vi "State Config.vi"(10 "stations count":i32=1, 11 "configuration file path":path) -> (0 "error out":errorcluster, 3 "all state configs":T4[](array[typedef]))   [LabVIEW 2018]
uses:
  Crl defs/DataStream.ctl
  Crl defs/one state paths config.ctl
  Crl defs/one state prints config.ctl
  Communication connection/Crl defs/print config.ctl
  Crl defs/one state scans config.ctl
  Communication connection/Crl defs/scanner config.ctl
  Crl defs/one state tags config.ctl
  Crl defs/PLC_bool tags.ctl
  DataSocket/Crl defs/DataSocket_Tags.ctl
  Crl defs/PLC_real tags.ctl
  Crl defs/PLC_string tags.ctl
  Crl defs/one state msic config.ctl
  Sequence/type defs/Sequence Info.ctl
  Crl defs/one state power supply config.ctl
  Crl defs/motor operating data.ctl
  Crl defs/one state screw config.ctl
  Crl defs/xls.data'S buffer.ctl
  Crl defs/XLS.header configs.ctl
  Interface/Crl defs/HomeScreens.ctl
  Interface/Crl defs/HomeScreen.ctl
  Interface/Crl defs/StatusBars.ctl
panel:
  out "HomeScreens":T1 {"Database LVDT's Data Out"."value" format="%.2f"; "StatusBar"."Cycle Time Br" format="%#_5g"}
  # "Pass / Fail"
  # "Station"
  # "Barcode"
  # "Barcode OK?"
  # "Ser Number"
  # "Part Type"
  # "Application Status"
  # "Cycle Time"
  # "Time"
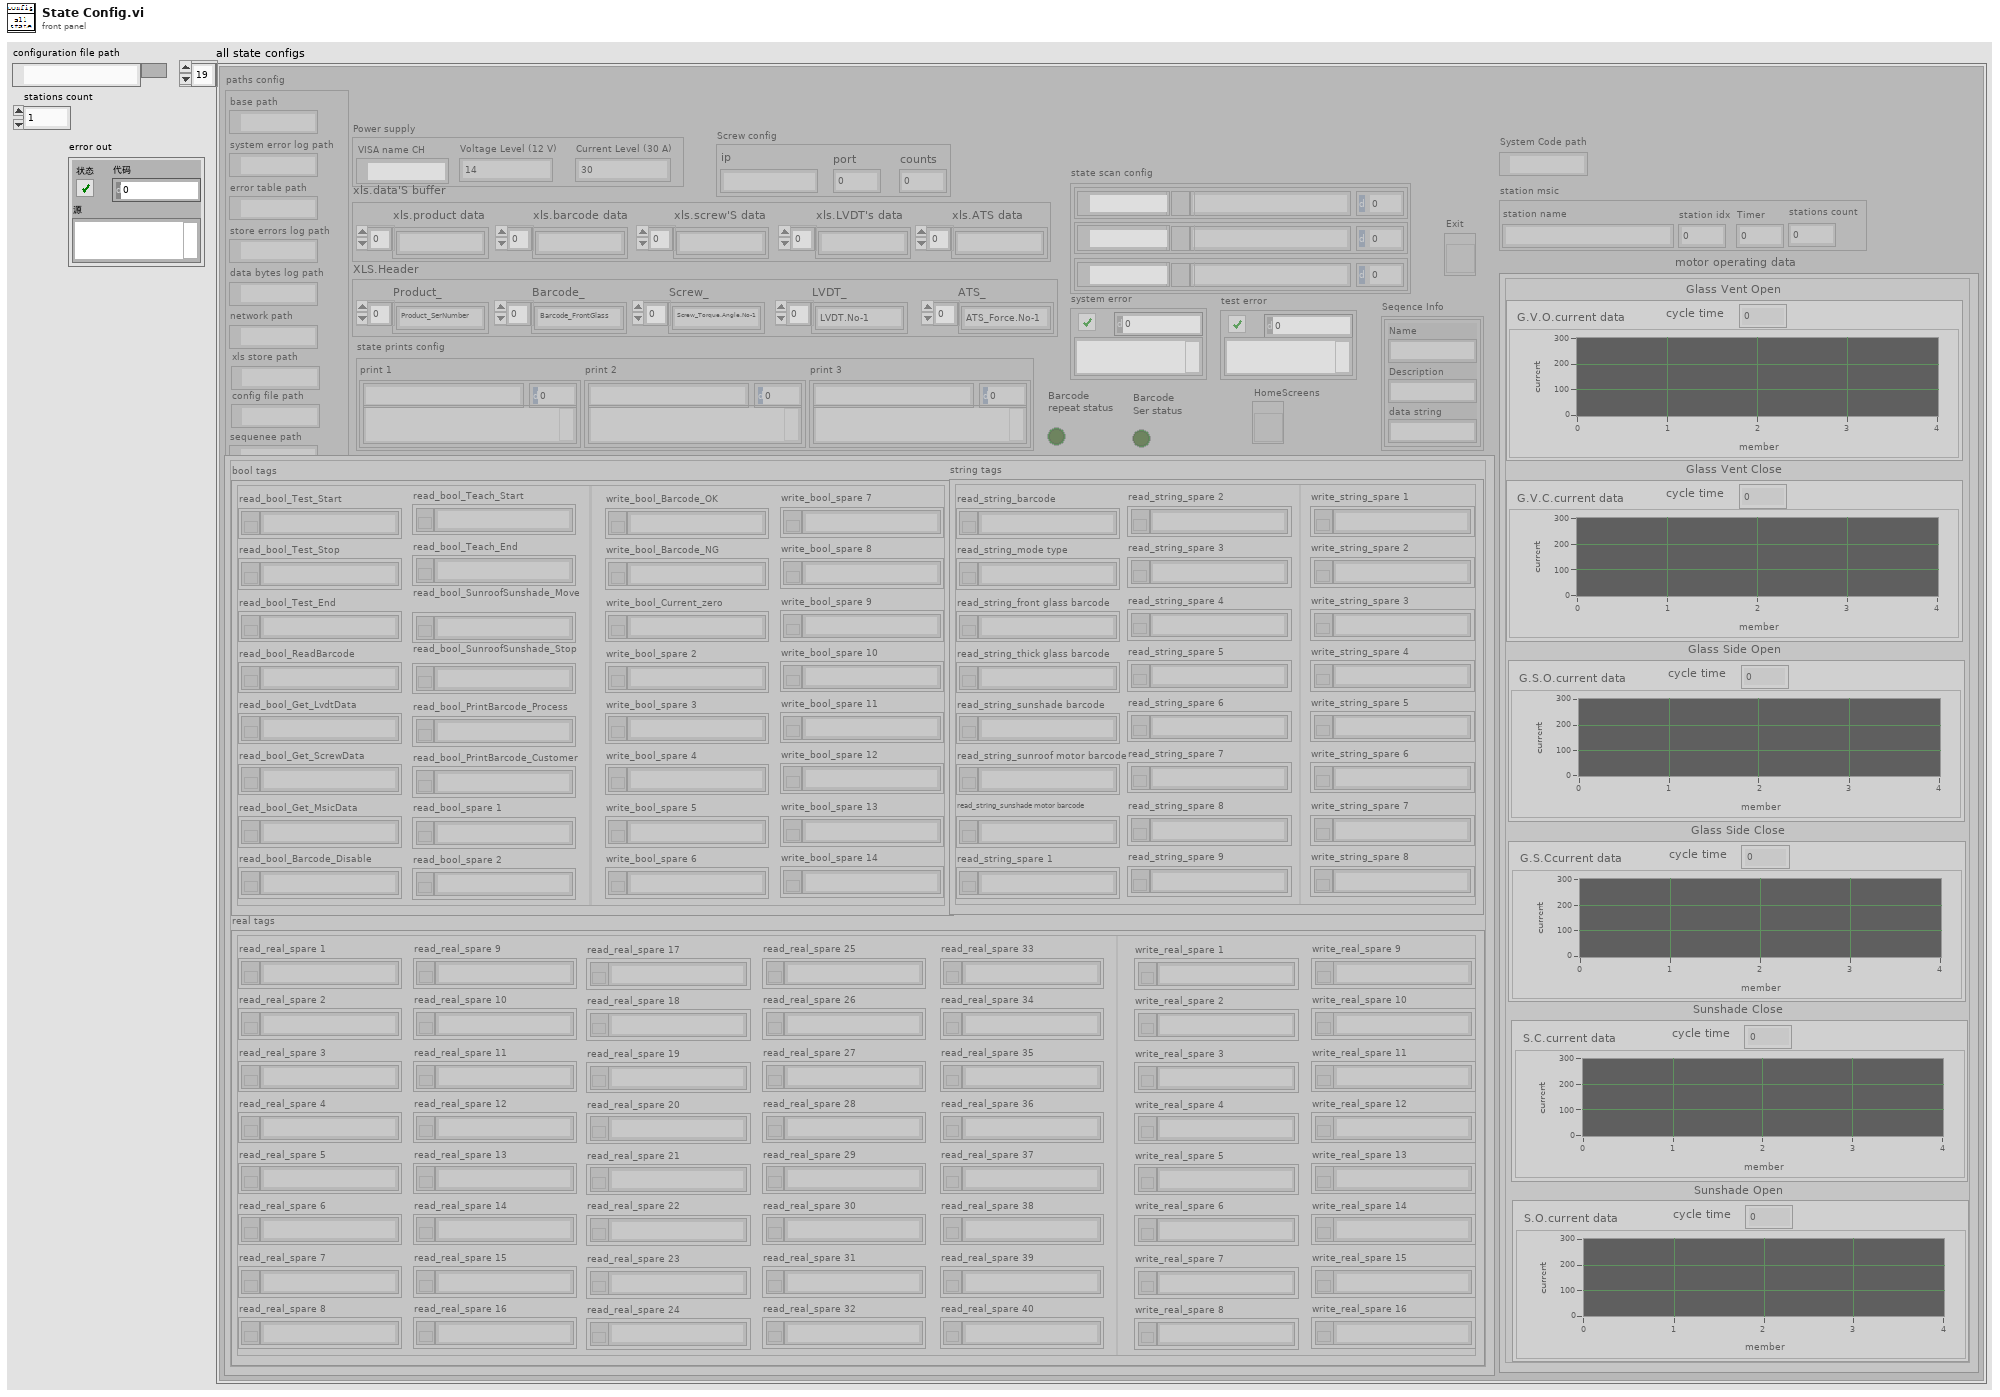
[diagram p1: front panel]
types:
  T1 = typedef "HomeScreens.ctl" = T2[]
  T2 = typedef "HomeScreen.ctl" = cluster{"StatusBar":T3, "Database LVDT's Data Out":cluster{"lvdt name":string, "value":dbl}[], "Screw.Data":string[], "Production information":string[][], "Error Table Br":string[][]}
  T3 = typedef "StatusBars.ctl" = cluster{"Station Name":string, "Barcode":string, "Ser Number":string, "Part Type":string, "Application Status":string, "Barcode Status":bool, "Pass / Fail":u32, "Cycle Time Br":dbl, "Time":string}
  T4 = typedef "DataStream.ctl" = cluster{"paths config":T5, "state prints config":T6, "state scan config":T8, "all tags of plc":T10, "station msic":T15, "test error":errorcluster, "system error":errorcluster, "Seqence Info":T16[], "Power supply":T17, "motor operating data":T18, "Screw config":T19, "xls.data'S buffer":T20, "XLS.Header":T21, "Barcode\nrepeat status":bool, "Barcode\nSer status":bool, "System Code path":path, "Exit":refnum<vi>, "HomeScreens":refnum<vi>}
  T5 = typedef "one state paths config.ctl" = cluster{"base path":path, "system error log path":path, "error table path":path, "store errors log path":path, "data bytes log path":path, "network path":path, "xls store path":path, "config file path":path, "sequenee path":path}
  T6 = typedef "one state prints config.ctl" = cluster{"print 1":T7, "print 2":T7, "print 3":T7}
  T7 = typedef "print config.ctl" = cluster{"connect ip or coms":string, "port":u16, "print strings":string}
  T8 = typedef "one state scans config.ctl" = cluster{"scan 1 ":T9, "scan 2":T9, "scan 3":T9}
  T9 = typedef "scanner config.ctl" = cluster{"connect ip or coms":string, "port":u16, "tcp connect id":refnum<k5>, "VISA resource name":refnum<visa-resource-name>}
  T10 = typedef "one state tags config.ctl" = cluster{"bool tags":T11, "real tags":T13, "string tags":T14}
  T11 = typedef "PLC_bool tags.ctl" = cluster{"read_bool_Test_Start":T12, "read_bool_Test_Stop":T12, "read_bool_Test_End":T12, "read_bool_ReadBarcode":T12, "read_bool_Get_LvdtData":T12, "read_bool_Get_ScrewData":T12, "read_bool_Get_MsicData":T12, "read_bool_Barcode_Disable":T12, "read_bool_Teach_Start":T12, "read_bool_Teach_End":T12, "read_bool_SunroofSunshade_Move":T12, "read_bool_SunroofSunshade_Stop":T12, "read_bool_PrintBarcode_Process":T12, "read_bool_PrintBarcode_Customer":T12, "read_bool_spare 1":T12, "read_bool_spare 2":T12, "write_bool_Barcode_OK":T12, "write_bool_Barcode_NG":T12, "write_bool_Current_zero":T12, "write_bool_spare 2":T12, "write_bool_spare 3":T12, "write_bool_spare 4":T12, "write_bool_spare 5":T12, "write_bool_spare 6":T12, "write_bool_spare 7":T12, "write_bool_spare 8":T12, "write_bool_spare 9":T12, "write_bool_spare 10":T12, "write_bool_spare 11":T12, "write_bool_spare 12":T12, "write_bool_spare 13":T12, "write_bool_spare 14":T12}
  T12 = typedef "DataSocket_Tags.ctl" = cluster{"Ds ID":refnum<k13>, "Tag":string}
  T13 = typedef "PLC_real tags.ctl" = cluster{"read_real_spare 1":T12, "read_real_spare 2":T12, "read_real_spare 3":T12, "read_real_spare 4":T12, "read_real_spare 5":T12, "read_real_spare 6":T12, "read_real_spare 7":T12, "read_real_spare 8":T12, "read_real_spare 9":T12, "read_real_spare 10":T12, "read_real_spare 11":T12, "read_real_spare 12":T12, "read_real_spare 13":T12, "read_real_spare 14":T12, "read_real_spare 15":T12, "read_real_spare 16":T12, "read_real_spare 17":T12, "read_real_spare 18":T12, "read_real_spare 19":T12, "read_real_spare 20":T12, "read_real_spare 21":T12, "read_real_spare 22":T12, "read_real_spare 23":T12, "read_real_spare 24":T12, "read_real_spare 25":T12, "read_real_spare 26":T12, "read_real_spare 27":T12, "read_real_spare 28":T12, "read_real_spare 29":T12, "read_real_spare 30":T12, "read_real_spare 31":T12, "read_real_spare 32":T12, "read_real_spare 33":T12, "read_real_spare 34":T12, "read_real_spare 35":T12, "read_real_spare 36":T12, "read_real_spare 37":T12, "read_real_spare 38":T12, "read_real_spare 39":T12, "read_real_spare 40":T12, "write_real_spare 1":T12, "write_real_spare 2":T12, "write_real_spare 3":T12, "write_real_spare 4":T12, "write_real_spare 5":T12, "write_real_spare 6":T12, "write_real_spare 7":T12, "write_real_spare 8":T12, "write_real_spare 9":T12, "write_real_spare 10":T12, "write_real_spare 11":T12, "write_real_spare 12":T12, "write_real_spare 13":T12, "write_real_spare 14":T12, "write_real_spare 15":T12, "write_real_spare 16":T12}
  T14 = typedef "PLC_string tags.ctl" = cluster{"read_string_barcode":T12, "read_string_mode type":T12, "read_string_front glass barcode":T12, "read_string_thick glass barcode":T12, "read_string_sunshade barcode":T12, "read_string_sunroof motor barcode":T12, "read_string_sunshade motor barcode\n":T12, "read_string_spare 1":T12, "read_string_spare 2":T12, "read_string_spare 3":T12, "read_string_spare 4":T12, "read_string_spare 5":T12, "read_string_spare 6":T12, "read_string_spare 7":T12, "read_string_spare 8":T12, "read_string_spare 9":T12, "write_string_spare 1":T12, "write_string_spare 2":T12, "write_string_spare 3":T12, "write_string_spare 4":T12, "write_string_spare 5":T12, "write_string_spare 6":T12, "write_string_spare 7":T12, "write_string_spare 8":T12}
  T15 = typedef "one state msic config.ctl" = cluster{"station name":string, "Timer":u32, "station idx":i32, "stations count":i32}
  T16 = typedef "Sequence Info.ctl" = cluster{"Name":string, "Description":string, "data string":string}
  T17 = typedef "one state power supply config.ctl" = cluster{"VISA name CH":refnum<visa-resource-name>, "Voltage Level (12 V)":dbl, "Current Level (30 A)":dbl}
  T18 = typedef "motor operating data.ctl" = cluster{"Glass Vent Open":cluster{"cycle time":sgl, "G.V.O.current data":sgl[]}, "Glass Vent Close":cluster{"cycle time":sgl, "G.V.C.current data":sgl[]}, "Glass Side Open":cluster{"cycle time":sgl, "G.S.O.current data":sgl[]}, "Glass Side Close":cluster{"cycle time":sgl, "G.S.Ccurrent data":sgl[]}, "Sunshade Close":cluster{"cycle time":sgl, "S.C.current data":sgl[]}, "Sunshade Open":cluster{"cycle time":sgl, "S.O.current data":sgl[]}}
  T19 = typedef "one state screw config.ctl" = cluster{"ip":string, "port":u16, "counts":u16}
  T20 = typedef "xls.data'S buffer.ctl" = cluster{"xls.product data":string[], "xls.barcode data":string[], "xls.screw'S data":string[], "xls.LVDT's data":string[], "xls.ATS data":string[]}
  T21 = typedef "XLS.header configs.ctl" = cluster{"Product_":string[], "Barcode_":string[], "Screw_":string[], "LVDT_":string[], "ATS_":string[]}
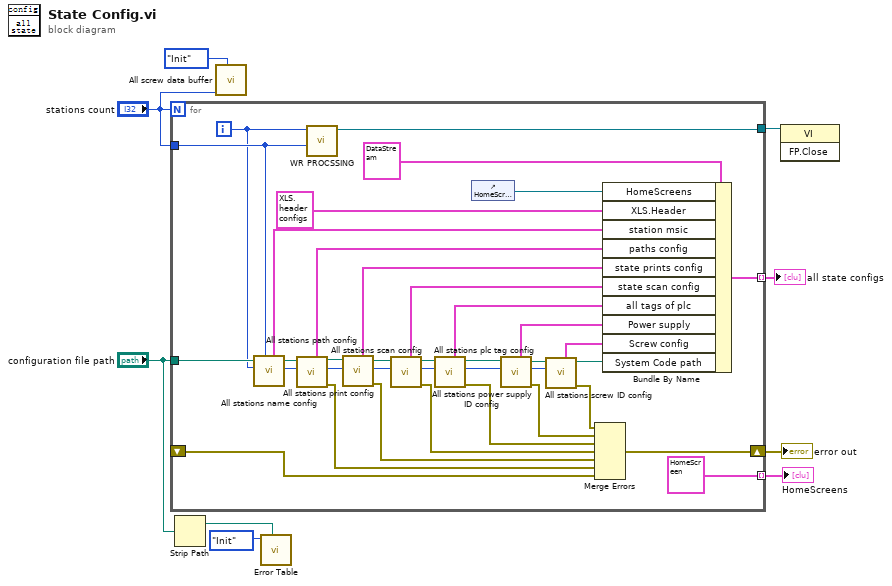
[diagram p0: block diagram]
diagram:
  n1 = for {
    N: "stations count" -> [_]
    shift-right: [w34] -> w9
    shift-left: _ -> [w33]
    tunnel: "configuration file path" -> [w31]
    tunnel: [w39] -> w3 mode=indexing
    tunnel: "stations count" -> [w16]
    tunnel: [w14] -> w7
    tunnel: [T2 {"StatusBar"={"Station Name"="", "Barcode"="", "Ser Number"="", "Part Type"="", "Application Status"="", "Barcode Status"=FALSE, "Pass / Fail"=9868950, "Cycle Time Br"=0.0, "Time"=""}, "Database LVDT's Data Out"=[], "Screw.Data"=[], "Production information"=[], "Error Table Br"=[]} ("HomeScreen")] -> w1 mode=indexing
    i -> [w15]
    n2 = call "All stations name config.vi"("stations count"=w16, "station idx"=w15, "configuration file path"=w31) -> ("station idx"=w25:i32, "configuration file path"=w32:path, "station msic"=w30:T15)  [unwired: 5 in, 1 out]
    n3 = call "All stations path config.vi"("station idx"=w25, "configuration file path"=w32) -> ("error out"=w35:errorcluster, "station idx"=w46:i32, "configuration file path"=w45:path, "paths config"=w43:T5)  [unwired: 6 in]
    n4 = call "WR PROCSSING.vi"("标尺.范围:最大值"=w16, "进度"=w15) -> ("本VI"=w14:refnum<vi>)  [unwired: 9 in]
    n5 = call "All stations print config.vi"("station idx"=w46, "configuration file path"=w45) -> ("error out"=w36:errorcluster, "station idx"=w29:i32, "configuration file path"=w28:path, "state prints config"=w42:T6)  [unwired: 6 in]
    n6 = call "All stations scan config.vi"("station idx"=w29, "configuration file path"=w28) -> ("error out"=w37:errorcluster, "station idx"=w26:i32, "configuration file path"=w27:path, "state scan config"=w41:T8)  [unwired: 6 in]
    n7 = call "All stations plc tag config.vi"("station idx"=w26, "configuration file path"=w27) -> ("error out"=w38:errorcluster, "station idx"=w23:i32, "configuration file path"=w24:path, "PLC Vaule"=w40:T10)  [unwired: 6 in]
    n8 = control-ref of="HomeScreens"() -> (w10:refnum<vi>)
    n9 = call "All stations power supply ID config.vi"("station idx"=w23, "configuration file path"=w24) -> ("error out"=w19:errorcluster, "station idx"=w20:i32, "configuration file path"=w21:path, "one state power supply"=w22:T17)  [unwired: 6 in]
    n10 = call "All stations screw ID config.vi"("station idx"=w20, "configuration file path"=w21) -> ("error out"=w18:errorcluster, "configuration file path"=w12:path, "Screw config"=w17:T19)  [unwired: 6 in, 1 out]
    n11 = Merge Errors(w18, w19, w38, w37, w36, w35, w33) -> (w34:errorcluster)
    n12 = Bundle By Name(cluster=T4 {"paths config"={"base path"=path "", "system error log path"=path "", "error table path"=path "", "store errors log path"=path "", "data bytes log path"=path "", "network path"=path "", "xls store path"=path "", "config file path"=path "", "sequenee path"=path ""}, "state prints config"={"print 1"={"connect ip or coms"="", "port"=0, "print strings"=""}, "print 2"={"connect ip or coms"="", "port"=0, "print strings"=""}, "print 3"={"connect ip or coms"="", "port"=0, "print strings"=""}}, "state scan config"={"scan 1 "={"connect ip or coms"="", "port"=0, "tcp connect id"=refnum, "VISA resource name"=""}, "scan 2"={"connect ip or coms"="", "port"=0, "tcp connect id"=refnum, "VISA resource name"=""}, "scan 3"={"connect ip or coms"="", "port"=0, "tcp connect id"=refnum, "VISA resource name"=""}}, "all tags of plc"={"bool tags"={"read_bool_Test_Start"={"Ds ID"=refnum, "Tag"=""}, "read_bool_Test_Stop"={"Ds ID"=refnum, "Tag"=""}, "read_bool_Test_End"={"Ds ID"=refnum, "Tag"=""}, "read_bool_ReadBarcode"={"Ds ID"=refnum, "Tag"=""}, "read_bool_Get_LvdtData"={"Ds ID"=refnum, "Tag"=""}, "read_bool_Get_ScrewData"={"Ds ID"=refnum, "Tag"=""}, "read_bool_Get_MsicData"={"Ds ID"=refnum, "Tag"=""}, "read_bool_Barcode_Disable"={"Ds ID"=refnum, "Tag"=""}, "read_bool_Teach_Start"={"Ds ID"=refnum, "Tag"=""}, "read_bool_Teach_End"={"Ds ID"=refnum, "Tag"=""}, "read_bool_SunroofSunshade_Move"={"Ds ID"=refnum, "Tag"=""}, "read_bool_SunroofSunshade_Stop"={"Ds ID"=refnum, "Tag"=""}, "read_bool_PrintBarcode_Process"={"Ds ID"=refnum, "Tag"=""}, "read_bool_PrintBarcode_Customer"={"Ds ID"=refnum, "Tag"=""}, "read_bool_spare 1"={"Ds ID"=refnum, "Tag"=""}, "read_bool_spare 2"={"Ds ID"=refnum, "Tag"=""}, "write_bool_Barcode_OK"={"Ds ID"=refnum, "Tag"=""}, "write_bool_Barcode_NG"={"Ds ID"=refnum, "Tag"=""}, "write_bool_Current_zero"={"Ds ID"=refnum, "Tag"=""}, "write_bool_spare 2"={"Ds ID"=refnum, "Tag"=""}, "write_bool_spare 3"={"Ds ID"=refnum, "Tag"=""}, "write_bool_spare 4"={"Ds ID"=refnum, "Tag"=""}, "write_bool_spare 5"={"Ds ID"=refnum, "Tag"=""}, "write_bool_spare 6"={"Ds ID"=refnum, "Tag"=""}, "write_bool_spare 7"={"Ds ID"=refnum, "Tag"=""}, "write_bool_spare 8"={"Ds ID"=refnum, "Tag"=""}, "write_bool_spare 9"={"Ds ID"=refnum, "Tag"=""}, "write_bool_spare 10"={"Ds ID"=refnum, "Tag"=""}, "write_bool_spare 11"={"Ds ID"=refnum, "Tag"=""}, "write_bool_spare 12"={"Ds ID"=refnum, "Tag"=""}, "write_bool_spare 13"={"Ds ID"=refnum, "Tag"=""}, "write_bool_spare 14"={"Ds ID"=refnum, "Tag"=""}}, "real tags"={"read_real_spare 1"={"Ds ID"=refnum, "Tag"=""}, "read_real_spare 2"={"Ds ID"=refnum, "Tag"=""}, "read_real_spare 3"={"Ds ID"=refnum, "Tag"=""}, "read_real_spare 4"={"Ds ID"=refnum, "Tag"=""}, "read_real_spare 5"={"Ds ID"=refnum, "Tag"=""}, "read_real_spare 6"={"Ds ID"=refnum, "Tag"=""}, "read_real_spare 7"={"Ds ID"=refnum, "Tag"=""}, "read_real_spare 8"={"Ds ID"=refnum, "Tag"=""}, "read_real_spare 9"={"Ds ID"=refnum, "Tag"=""}, "read_real_spare 10"={"Ds ID"=refnum, "Tag"=""}, "read_real_spare 11"={"Ds ID"=refnum, "Tag"=""}, "read_real_spare 12"={"Ds ID"=refnum, "Tag"=""}, "read_real_spare 13"={"Ds ID"=refnum, "Tag"=""}, "read_real_spare 14"={"Ds ID"=refnum, "Tag"=""}, "read_real_spare 15"={"Ds ID"=refnum, "Tag"=""}, "read_real_spare 16"={"Ds ID"=refnum, "Tag"=""}, "read_real_spare 17"={"Ds ID"=refnum, "Tag"=""}, "read_real_spare 18"={"Ds ID"=refnum, "Tag"=""}, "read_real_spare 19"={"Ds ID"=refnum, "Tag"=""}, "read_real_spare 20"={"Ds ID"=refnum, "Tag"=""}, "read_real_spare 21"={"Ds ID"=refnum, "Tag"=""}, "read_real_spare 22"={"Ds ID"=refnum, "Tag"=""}, "read_real_spare 23"={"Ds ID"=refnum, "Tag"=""}, "read_real_spare 24"={"Ds ID"=refnum, "Tag"=""}, "read_real_spare 25"={"Ds ID"=refnum, "Tag"=""}, "read_real_spare 26"={"Ds ID"=refnum, "Tag"=""}, "read_real_spare 27"={"Ds ID"=refnum, "Tag"=""}, "read_real_spare 28"={"Ds ID"=refnum, "Tag"=""}, "read_real_spare 29"={"Ds ID"=refnum, "Tag"=""}, "read_real_spare 30"={"Ds ID"=refnum, "Tag"=""}, "read_real_spare 31"={"Ds ID"=refnum, "Tag"=""}, "read_real_spare 32"={"Ds ID"=refnum, "Tag"=""}, "read_real_spare 33"={"Ds ID"=refnum, "Tag"=""}, "read_real_spare 34"={"Ds ID"=refnum, "Tag"=""}, "read_real_spare 35"={"Ds ID"=refnum, "Tag"=""}, "read_real_spare 36"={"Ds ID"=refnum, "Tag"=""}, "read_real_spare 37"={"Ds ID"=refnum, "Tag"=""}, "read_real_spare 38"={"Ds ID"=refnum, "Tag"=""}, "read_real_spare 39"={"Ds ID"=refnum, "Tag"=""}, "read_real_spare 40"={"Ds ID"=refnum, "Tag"=""}, "write_real_spare 1"={"Ds ID"=refnum, "Tag"=""}, "write_real_spare 2"={"Ds ID"=refnum, "Tag"=""}, "write_real_spare 3"={"Ds ID"=refnum, "Tag"=""}, "write_real_spare 4"={"Ds ID"=refnum, "Tag"=""}, "write_real_spare 5"={"Ds ID"=refnum, "Tag"=""}, "write_real_spare 6"={"Ds ID"=refnum, "Tag"=""}, "write_real_spare 7"={"Ds ID"=refnum, "Tag"=""}, "write_real_spare 8"={"Ds ID"=refnum, "Tag"=""}, "write_real_spare 9"={"Ds ID"=refnum, "Tag"=""}, "write_real_spare 10"={"Ds ID"=refnum, "Tag"=""}, "write_real_spare 11"={"Ds ID"=refnum, "Tag"=""}, "write_real_spare 12"={"Ds ID"=refnum, "Tag"=""}, "write_real_spare 13"={"Ds ID"=refnum, "Tag"=""}, "write_real_spare 14"={"Ds ID"=refnum, "Tag"=""}, "write_real_spare 15"={"Ds ID"=refnum, "Tag"=""}, "write_real_spare 16"={"Ds ID"=refnum, "Tag"=""}}, "string tags"={"read_string_barcode"={"Ds ID"=refnum, "Tag"=""}, "read_string_mode type"={"Ds ID"=refnum, "Tag"=""}, "read_string_front glass barcode"={"Ds ID"=refnum, "Tag"=""}, "read_string_thick glass barcode"={"Ds ID"=refnum, "Tag"=""}, "read_string_sunshade barcode"={"Ds ID"=refnum, "Tag"=""}, "read_string_sunroof motor barcode"={"Ds ID"=refnum, "Tag"=""}, "read_string_sunshade motor barcode\n"={"Ds ID"=refnum, "Tag"=""}, "read_string_spare 1"={"Ds ID"=refnum, "Tag"=""}, "read_string_spare 2"={"Ds ID"=refnum, "Tag"=""}, "read_string_spare 3"={"Ds ID"=refnum, "Tag"=""}, "read_string_spare 4"={"Ds ID"=refnum, "Tag"=""}, "read_string_spare 5"={"Ds ID"=refnum, "Tag"=""}, "read_string_spare 6"={"Ds ID"=refnum, "Tag"=""}, "read_string_spare 7"={"Ds ID"=refnum, "Tag"=""}, "read_string_spare 8"={"Ds ID"=refnum, "Tag"=""}, "read_string_spare 9"={"Ds ID"=refnum, "Tag"=""}, "write_string_spare 1"={"Ds ID"=refnum, "Tag"=""}, "write_string_spare 2"={"Ds ID"=refnum, "Tag"=""}, "write_string_spare 3"={"Ds ID"=refnum, "Tag"=""}, "write_string_spare 4"={"Ds ID"=refnum, "Tag"=""}, "write_string_spare 5"={"Ds ID"=refnum, "Tag"=""}, "write_string_spare 6"={"Ds ID"=refnum, "Tag"=""}, "write_string_spare 7"={"Ds ID"=refnum, "Tag"=""}, "write_string_spare 8"={"Ds ID"=refnum, "Tag"=""}}}, "station msic"={"station name"="", "Timer"=0, "station idx"=0, "stations count"=0}, "test error"={"status"=FALSE, "code"=0, "source"=""}, "system error"={"status"=FALSE, "code"=0, "source"=""}, "Seqence Info"=[], "Power supply"={"VISA name CH"="", "Voltage Level (12 V)"=0.0, "Current Level (30 A)"=0.0}, "motor operating data"={"Glass Vent Open"={"cycle time"=0.0, "G.V.O.current data"=[]}, "Glass Vent Close"={"cycle time"=0.0, "G.V.C.current data"=[]}, "Glass Side Open"={"cycle time"=0.0, "G.S.O.current data"=[]}, "Glass Side Close"={"cycle time"=0.0, "G.S.Ccurrent data"=[]}, "Sunshade Close"={"cycle time"=0.0, "S.C.current data"=[]}, "Sunshade Open"={"cycle time"=0.0, "S.O.current data"=[]}}, "Screw config"={"ip"="", "port"=0, "counts"=0}, "xls.data'S buffer"={"xls.product data"=[], "xls.barcode data"=[], "xls.screw'S data"=[], "xls.LVDT's data"=[], "xls.ATS data"=[]}, "XLS.Header"={"Product_"=[], "Barcode_"=[], "Screw_"=[], "LVDT_"=[], "ATS_"=[]}, "Barcode\nrepeat status"=FALSE, "Barcode\nSer status"=FALSE, "System Code path"=path "", "Exit"=refnum, "HomeScreens"=refnum} ("all state configs"), "HomeScreens"=w10, "XLS.Header"=T21 {"Product_"=["Product_SerNumber", "Product_Time", "Product_ModeType", "Product_ProcessBarcode", "Product_CycleTmie"], "Barcode_"=["Barcode_FrontGlass", "Barcode_RearGlass", "Barcode_Sunshade", "Barcode_SunroofMotor", "Barcode_SunshadeMotor", "Barcode_FrontBeam", "Barcode_RearBeam", "Barcode_LeftGuideRail", "Barcode_RightGuideRail"], "Screw_"=["Screw_Torque.Angle.No-1", "Screw_Torque.Angle.No-2", "Screw_Torque.Angle.No-3", "Screw_Torque.Angle.No-4", "Screw_Torque.Angle.No-5", "Screw_Torque.Angle.No-6", "Screw_Torque.Angle.No-7", "Screw_Torque.Angle.No-8", "Screw_Torque.Angle.No-9", "Screw_Torque.Angle.No-10", "Screw_Torque.Angle.No-11", "Screw_Torque.Angle.No-12"], "LVDT_"=["LVDT.No-1", "LVDT.No-2", "LVDT.No-3", "LVDT.No-4", "LVDT.No-5", "LVDT.No-6", "LVDT.No-7", "LVDT.No-8", "LVDT.No-9", "LVDT.No-10", "LVDT.No-11", "LVDT.No-12", "LVDT.No-13", "LVDT.No-14", "LVDT.No-15", "LVDT.No-16", "LVDT.No-17", "LVDT.No-18", "LVDT.No-19", "LVDT.No-20"], "ATS_"=["ATS_Force.No-1", "ATS_Force.No-2", "ATS_Force.No-3", "ATS_Force.No-4"]}, "station msic"=w30, "paths config"=w43, "state prints config"=w42, "state scan config"=w41, "all tags of plc"=w40, "Power supply"=w22, "Screw config"=w17, "System Code path"=w12) -> (w39:T4)
  }
  "error out" <- w9
  "all state configs" <- w3
  "HomeScreens" <- w1
  n13 = Strip Path(path="configuration file path") -> (stripped path=w5:path)  [unwired: 1 out]
  n14 = call "All screw data buffer.vi"("Mode"=enum16{"Read", "Write", "Error", "Init"}."Init", "station counts"="stations count") -> ()  [unwired: 4 in, 6 out]
  n15 = call "Error Table.vi"("Path"=w5, "Error Mode"=enum16{"Init", "Get Error"}."Init") -> ()  [unwired: 8 in, 2 out]
  n16 = invoke class="VI" method="FP.Close"(reference=w7) -> ()  [unwired: 2 in, 3 out]
